vi "Set Acceleration.vi"(8 "error in (no error)":errorcluster, 10 "Acceleration":dbl, 11 "SIM Motion Controller in":refnum<class "Fine SIM Motion Controller.lvclass">) -> (0 "error out":errorcluster, 3 "SIM Motion Controller out":refnum<class "Fine SIM Motion Controller.lvclass">)   [LabVIEW 2022 SP3, in "Fine SIM Motion Controller.lvclass"]
uses:
  Fine SIM Motion Controller.lvclass
  Fine SIM Motion Controller.lvclass/Fine SIM Motion Controller.ctl
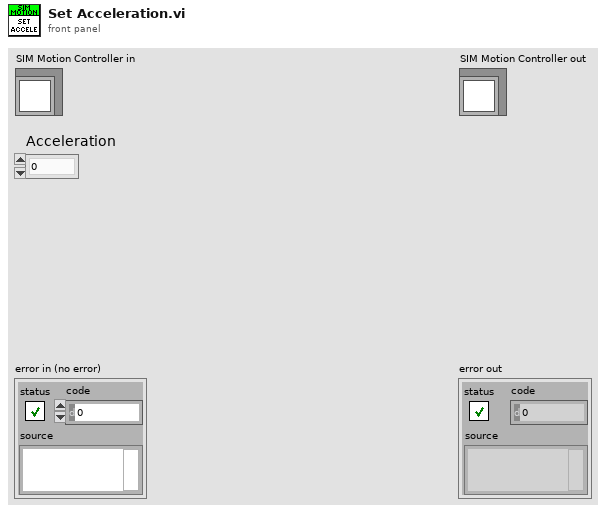
[diagram p1: front panel]
types:
  T1 = typedef "Parent SIM Motion Controller.lvclass/Axis Data.ctl" = cluster{"Axis Parameters":T2, "Axis Settings":T3, "Time Stamp":timestamp}
  T2 = typedef "Parent SIM Motion Controller.lvclass/Axis Parameters.ctl" = cluster{"Moving":bool, "Homed":bool, "Desired Position":dbl, "Current Positon":dbl, "Current Speed":dbl}
  T3 = typedef "Parent SIM Motion Controller.lvclass/Axis Settings.ctl" = cluster{"Speed":dbl, "Acceleration":dbl}
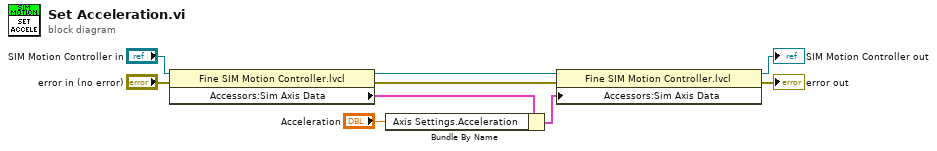
[diagram p0: block diagram]
diagram:
  n1 = property class="Fine SIM Motion Controller.lvcl"(reference="SIM Motion Controller in", error in="error in (no error)") -> (reference out=w8:refnum<class "Fine SIM Motion Controller.lvclass">, error out=w3:errorcluster, "Accessors:Sim Axis Data"=w2:T1)
  n2 = Bundle By Name(cluster=w2, "Axis Settings.Acceleration"="Acceleration") -> (w1:T1)
  n3 = property class="Fine SIM Motion Controller.lvcl"(reference=w8, error in=w3, "Accessors:Sim Axis Data"=w1) -> (reference out=→"SIM Motion Controller out":refnum<class "Fine SIM Motion Controller.lvclass">, error out=→"error out":errorcluster)
